vi "FPGA Read By Name - Boolean.vi"(8 "error in (no error)":errorcluster, 10 "Indicator":string, 11 "FPGA Session In":refnum<class "FPGA Interface Base.lvclass">) -> (0 "error out":errorcluster, 2 "Value":bool, 3 "FPGA Session Out":refnum<class "FPGA Interface Base.lvclass">)   [LabVIEW 2010, in "FPGA Interface Base.lvclass"]
doc: "Reads a boolean value from a given indicator or control."
uses:
  <userlib>/_FPGA Interface Advanced Tools/FPGA Interface Base/FPGA Interface Base.lvclass
  <vilib>/rvi/DataTransferAndStorage/Container/Common/niFpgaDataTypeControl.ctl
  <userlib>/_FPGA Interface Advanced Tools/FPGA Interface Base/FPGA Interface Base.lvclass/FPGA Interface Base.ctl
  <vilib>/Utility/error.llb/Error Cluster From Error Code.vi
  <userlib>/_FPGA Interface Advanced Tools/FPGA Interface Base/Accessors/FPGA Read Session.vi
  <userlib>/_FPGA Interface Advanced Tools/FPGA Interface Wrapper/FPGA Interface Wrapper.lvlib
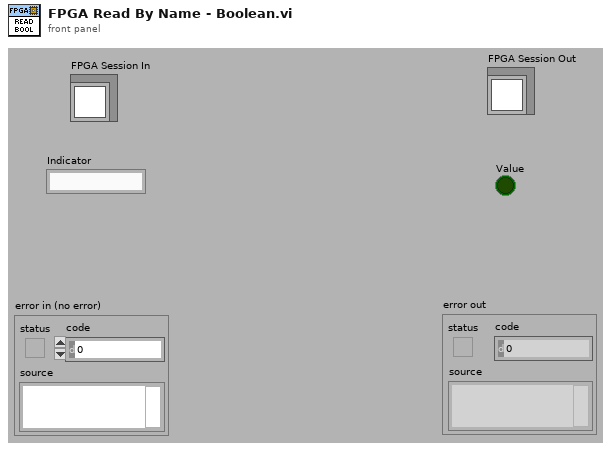
[diagram p1: front panel]
types:
  T1 = typedef "niFpgaDataTypeControl.ctl" = enum32{"Boolean", "I8", "I16", "I32", "I64", "U8", "U16", "U32", "U64", "FXP", "CustomControl"}
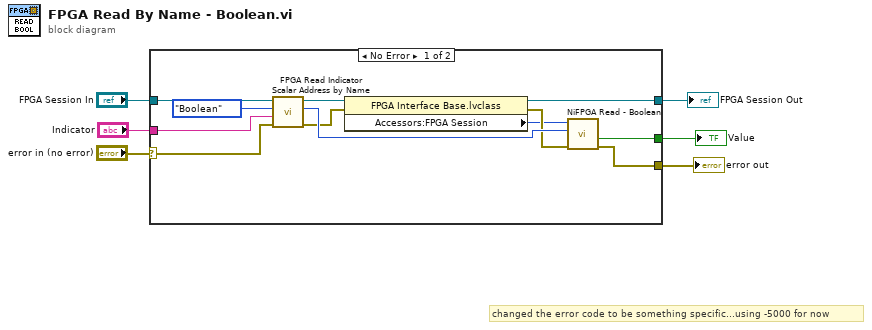
[diagram p0: block diagram]
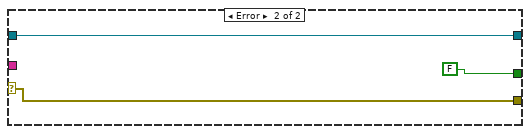
[diagram p2: hidden frame]
diagram:
  # "changed the error code to be something specific...using -5000 for now"
  n1 = case shown="No Error" "error in (no error)" {
    selector: "error in (no error)" -> [w10 w21]
    tunnel: [w8 w21] -> w5
    tunnel: [w9 w19] -> w2
    tunnel: [w18 FALSE] -> w4
    tunnel: "FPGA Session In" -> [w11 w19]
    tunnel: "Indicator" -> [w7 _]
    frame No Error {
      n2 = call <userlib>:"FPGA Read Indicator Scalar Address by Name.vi"("error in (no error)"=w10, "Name"=w7, "Data Type"=niFpgaDataTypeControl."Boolean", "FPGA Interface Base in"=w11) -> ("error out"=w15:errorcluster, "Address"=w16:u32, "FPGA Interface Base out"=w14:refnum<class "FPGA Interface Base.lvclass">)  [unwired: 4 in, 1 out]
      n3 = property class="FPGA Interface Base.lvclass"(reference=w14, error in=w15) -> (reference out=w9:refnum<class "FPGA Interface Base.lvclass">, error out=w13:errorcluster, "Accessors:FPGA Session"=w12:u32)
      n4 = call <userlib>:"NiFPGA Read - Boolean.vi"("error in (no error)"=w13, "Indicator"=w16, "Session"=w12) -> ("error out"=w8:errorcluster, "Boolean"=w18:bool)  [unwired: 6 in, 1 out]
    }
    frame Error {
    }
  }
  "error out" <- w5
  "Value" <- w4
  "FPGA Session Out" <- w2
